vi "ExportCallback.vi"(4 "GetV5Instance":refnum<k24>, 6 "Control Ref":refnum<k24>, 7 "Event Common Data":T2) -> ()   [LabVIEW 2010]
uses:
  C:/Program Files/Spiricon/BeamGage Enterprise/Spiricon.BeamGage.Automation.dll
  Program Files/Spiricon/BeamGage Enterprise/Spiricon.BeamGage.Automation.dll
  C:/Program Files/Spiricon/BeamGage Enterprise/Spiricon.BeamGage.Automation.Interfaces.dll
  Program Files/Spiricon/BeamGage Enterprise/Spiricon.BeamGage.Automation.Interfaces.dll
panel:
  out "AExportStatusEnum":T1(ring)
  out "AExportStatus":i32
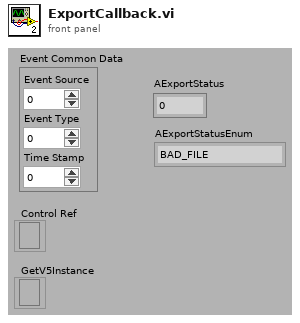
[diagram p1: front panel]
types:
  T1 = enum16{"BAD_FILE", "BAD_FRAME_NUM", "BASE_FILE_EXISTS", "BASE_FILE_IS_DIRECTORY", "GOOD", "NO_FILE_NAME", "NO_IMAGE", "READ_ONLY"}
  T2 = cluster{"Event Source":i32, "Event Type":u32, "Time Stamp":u32}
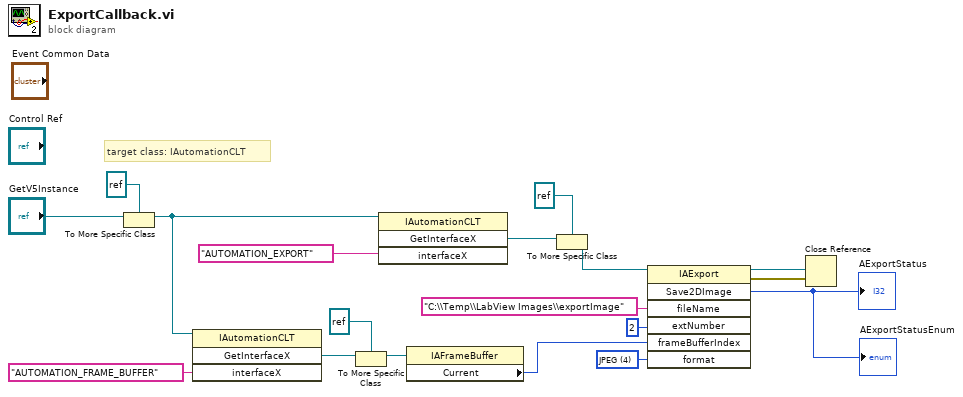
[diagram p0: block diagram]
diagram:
  w13 = 4 items=["NONE", "ASCII", "BMP", "GIF", "JPEG", "PNG", "TIFF"] ("format")
  # "target class: IAutomationCLT"
  n1 = To More Specific Class(target class=refnum<k24> refnum, reference="GetV5Instance") -> (specific class reference=w5:refnum<k24>)  [unwired: 1 in, 1 out]
  n2 = invoke class="IAutomationCLT" method="GetInterfaceX"(reference=w5, "interfaceX"="AUTOMATION_FRAME_BUFFER") -> ("GetInterfaceX"=w9:refnum<k24>)  [unwired: 2 in, 3 out]
  n3 = To More Specific Class(target class=refnum<k24> refnum, reference=w9) -> (specific class reference=w7:refnum<k24>)  [unwired: 1 in, 1 out]
  n4 = invoke class="IAutomationCLT" method="GetInterfaceX"(reference=w5, "interfaceX"="AUTOMATION_EXPORT") -> ("GetInterfaceX"=w11:refnum<k24>)  [unwired: 2 in, 3 out]
  n5 = property class="IAFrameBuffer"(reference=w7) -> ("Current"=w6:u32)  [unwired: 1 in, 2 out]
  n6 = To More Specific Class(target class=refnum<k24> refnum, reference=w11) -> (specific class reference=w16:refnum<k24>)  [unwired: 1 in, 1 out]
  n7 = invoke class="IAExport" method="Save2DImage"(reference=w16, "fileName"="C:\\Temp\\LabView Images\\exportImage", "extNumber"=u32 2, "frameBufferIndex"=w6, "format"=w13) -> (reference out=w15:refnum<k24>, error out=w14:errorcluster, "Save2DImage"=→"AExportStatus" →"AExportStatusEnum":i32)  [unwired: 2 in, 4 out]
  n8 = Close Reference(reference=w15, error in (no error)=w14) -> ()  [unwired: 1 out]
